vi "Write Action.vi"(8 "error in (no error)":errorcluster, 10 "Action":string, 11 "Action in":refnum<class "Action.lvclass">) -> (0 "error out":errorcluster, 3 "Action out":refnum<class "Action.lvclass">)   [LabVIEW 2013, in "Messages.lvlib" / "Action.lvclass"]
uses:
  Action.lvclass
  Action.lvclass/Action.ctl
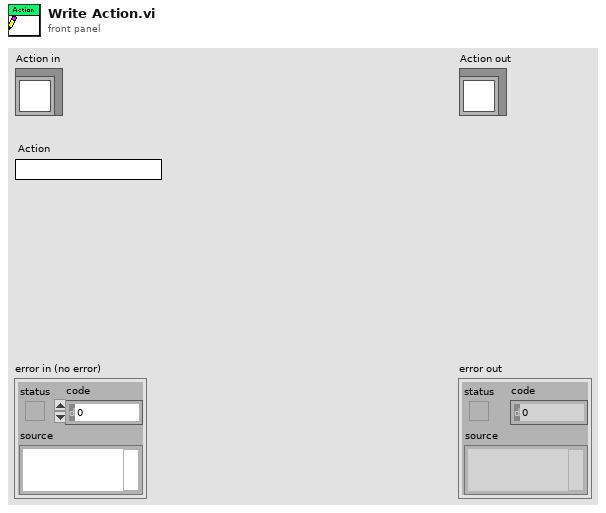
[diagram p1: front panel]
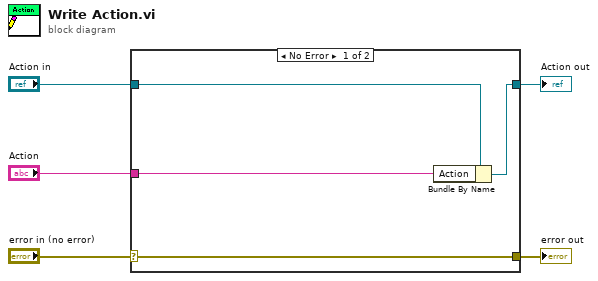
[diagram p0: block diagram]
diagram:
  n1 = case shown="No Error" "error in (no error)" {
    selector: "error in (no error)" -> [w9 w10]
    tunnel: [w9 w10] -> w4
    tunnel: [w7 w11] -> w2
    tunnel: "Action in" -> [w8 w11]
    tunnel: "Action" -> [w6 _]
    frame No Error {
      n2 = Bundle By Name(cluster=w8, "Action"=w6) -> (w7:refnum<class "Action.lvclass">)
    }
    frame Error {
    }
  }
  "error out" <- w4
  "Action out" <- w2
